vi "AnalogDemultiplex_AND_drop_first_sample.vi"(0 "Analog data cluster":T1, 11 "Last? Input":bool) -> (4 "Data A1 out":u64, 6 "Data A2 out":u64, 15 "Last? Output":bool)   [LabVIEW 2012]
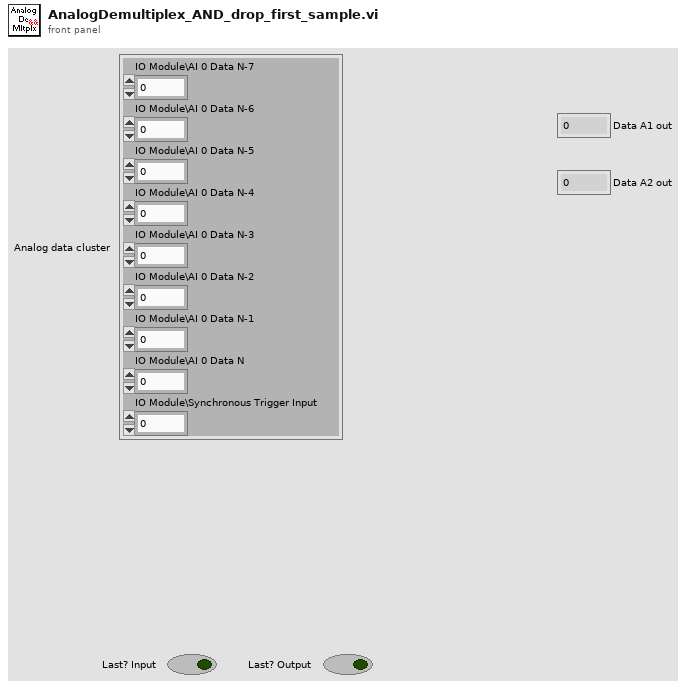
[diagram p1: front panel]
types:
  T1 = cluster{"IO Module\\AI 0 Data N-7":u8, "IO Module\\AI 0 Data N-6":u8, "IO Module\\AI 0 Data N-5":u8, "IO Module\\AI 0 Data N-4":u8, "IO Module\\AI 0 Data N-3":u8, "IO Module\\AI 0 Data N-2":u8, "IO Module\\AI 0 Data N-1":u8, "IO Module\\AI 0 Data N":u8, "IO Module\\Synchronous Trigger Input":u8}
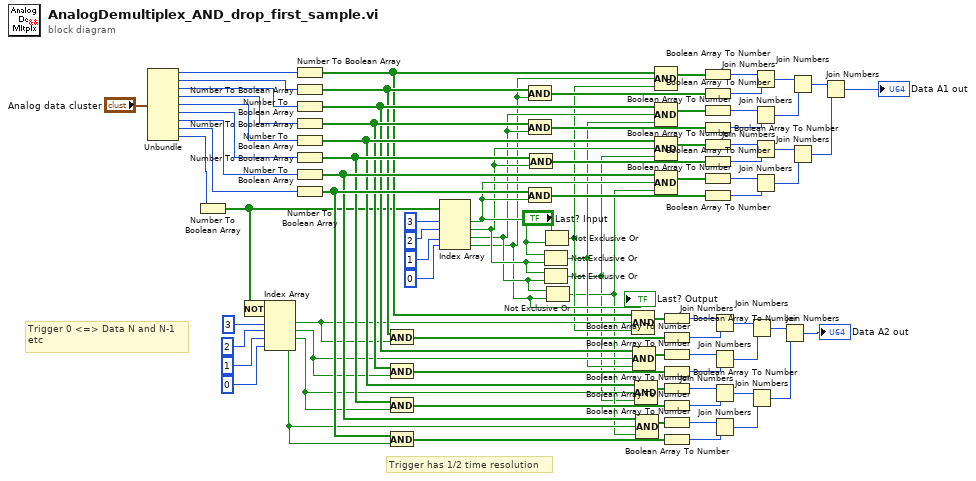
[diagram p0: block diagram]
diagram:
  # "Trigger 0 <=> Data N and N-1\netc"
  # "Trigger has 1/2 time resolution"
  n1 = Unbundle("Analog data cluster") -> ("IO Module\\AI 0 Data N-7"=w27:u8, "IO Module\\AI 0 Data N-6"=w26:u8, "IO Module\\AI 0 Data N-5"=w25:u8, "IO Module\\AI 0 Data N-4"=w24:u8, "IO Module\\AI 0 Data N-3"=w23:u8, "IO Module\\AI 0 Data N-2"=w22:u8, "IO Module\\AI 0 Data N-1"=w21:u8, "IO Module\\AI 0 Data N"=w20:u8, "IO Module\\Synchronous Trigger Input"=w19:u8)
  n2 = Number To Boolean Array(number=w19) -> (Boolean array=w50:bool[])
  n3 = Not(x=w50) -> (.not. x?=w51:bool[])
  n4 = Index Array(array=w51, index #1=3 ("index"), index #2=2 ("index"), index #3=1 ("index"), index #4=0 ("index")) -> (element #1=w66:bool, element #2=w67:bool, element #3=w68:bool, element #4=w69:bool)
  n5 = Number To Boolean Array(number=w27) -> (Boolean array=w70:bool[])
  n6 = Number To Boolean Array(number=w26) -> (Boolean array=w71:bool[])
  n7 = Number To Boolean Array(number=w25) -> (Boolean array=w72:bool[])
  n8 = Number To Boolean Array(number=w24) -> (Boolean array=w73:bool[])
  n9 = Number To Boolean Array(number=w23) -> (Boolean array=w74:bool[])
  n10 = Number To Boolean Array(number=w22) -> (Boolean array=w75:bool[])
  n11 = Number To Boolean Array(number=w21) -> (Boolean array=w76:bool[])
  n12 = Number To Boolean Array(number=w20) -> (Boolean array=w77:bool[])
  n13 = And(x=w71, y=w66) -> (x .and. y?=w79:bool[])
  n14 = And(x=w73, y=w67) -> (x .and. y?=w81:bool[])
  n15 = And(x=w75, y=w68) -> (x .and. y?=w83:bool[])
  n16 = And(x=w77, y=w69) -> (x .and. y?=w85:bool[])
  n17 = Index Array(array=w50, index #1=3 ("index"), index #2=2 ("index"), index #3=1 ("index"), index #4=0 ("index")) -> (element #1=w8:bool, element #2=w7:bool, element #3=w6:bool, element #4=w5:bool)
  "Last? Output" <- w5
  n18 = And(x=w71, y=w5) -> (x .and. y?=w36:bool[])
  n19 = And(x=w73, y=w6) -> (x .and. y?=w38:bool[])
  n20 = And(x=w77, y=w8) -> (x .and. y?=w42:bool[])
  n21 = And(x=w75, y=w7) -> (x .and. y?=w40:bool[])
  n22 = Not Exclusive Or(1:w7, 2:w8) -> (0:w3:bool)
  n23 = Not Exclusive Or(1:w6, 2:w7) -> (0:w1:bool)
  n24 = Not Exclusive Or(1:w8, 2:"Last? Input") -> (0:w4:bool)
  n25 = Not Exclusive Or(1:w5, 2:w6) -> (0:w2:bool)
  n26 = Compound Arithmetic op=AND(w70, w66, w4) -> (w78:bool[])
  n27 = Compound Arithmetic op=AND(w72, w67, w3) -> (w80:bool[])
  n28 = Compound Arithmetic op=AND(w74, w68, w1) -> (w82:bool[])
  n29 = Compound Arithmetic op=AND(w76, w69, w2) -> (w84:bool[])
  n30 = Compound Arithmetic op=AND(w70, w5, w4) -> (w34:bool[])
  n31 = Compound Arithmetic op=AND(w72, w6, w3) -> (w37:bool[])
  n32 = Compound Arithmetic op=AND(w74, w7, w1) -> (w39:bool[])
  n33 = Compound Arithmetic op=AND(w76, w8, w2) -> (w41:bool[])
  n34 = Boolean Array To Number(Boolean array=w78) -> (number=w58:u8)
  n35 = Boolean Array To Number(Boolean array=w79) -> (number=w59:u8)
  n36 = Boolean Array To Number(Boolean array=w80) -> (number=w60:u8)
  n37 = Boolean Array To Number(Boolean array=w81) -> (number=w61:u8)
  n38 = Boolean Array To Number(Boolean array=w82) -> (number=w62:u8)
  n39 = Boolean Array To Number(Boolean array=w83) -> (number=w63:u8)
  n40 = Boolean Array To Number(Boolean array=w84) -> (number=w64:u8)
  n41 = Boolean Array To Number(Boolean array=w85) -> (number=w65:u8)
  n42 = Boolean Array To Number(Boolean array=w34) -> (number=w35:u8)
  n43 = Boolean Array To Number(Boolean array=w36) -> (number=w43:u8)
  n44 = Boolean Array To Number(Boolean array=w37) -> (number=w44:u8)
  n45 = Boolean Array To Number(Boolean array=w38) -> (number=w45:u8)
  n46 = Boolean Array To Number(Boolean array=w39) -> (number=w46:u8)
  n47 = Boolean Array To Number(Boolean array=w40) -> (number=w47:u8)
  n48 = Boolean Array To Number(Boolean array=w41) -> (number=w48:u8)
  n49 = Boolean Array To Number(Boolean array=w42) -> (number=w49:u8)
  n50 = Join Numbers(hi=w58, lo=w59) -> ((hi.lo)=w52:u16)
  n51 = Join Numbers(hi=w60, lo=w61) -> ((hi.lo)=w53:u16)
  n52 = Join Numbers(hi=w62, lo=w63) -> ((hi.lo)=w54:u16)
  n53 = Join Numbers(hi=w64, lo=w65) -> ((hi.lo)=w55:u16)
  n54 = Join Numbers(hi=w52, lo=w53) -> ((hi.lo)=w57:u32)
  n55 = Join Numbers(hi=w54, lo=w55) -> ((hi.lo)=w56:u32)
  n56 = Join Numbers(hi=w35, lo=w43) -> ((hi.lo)=w28:u16)
  n57 = Join Numbers(hi=w44, lo=w45) -> ((hi.lo)=w29:u16)
  n58 = Join Numbers(hi=w46, lo=w47) -> ((hi.lo)=w30:u16)
  n59 = Join Numbers(hi=w48, lo=w49) -> ((hi.lo)=w31:u16)
  n60 = Join Numbers(hi=w57, lo=w56) -> ((hi.lo)=→"Data A2 out":u64)
  n61 = Join Numbers(hi=w28, lo=w29) -> ((hi.lo)=w33:u32)
  n62 = Join Numbers(hi=w30, lo=w31) -> ((hi.lo)=w32:u32)
  n63 = Join Numbers(hi=w33, lo=w32) -> ((hi.lo)=→"Data A1 out":u64)
